vi "2D&3D Trajectory.vi"() -> ()   [LabVIEW 2014]
uses:
  <vilib>/LVH/AR Drone Toolkit/Decode NavData/Typedefs/NavData Demo.ctl
  <vilib>/Native 3D Graph/xcontrol/3DPC_SurfacePlot.xctl
  <vilib>/LVH/AR Drone Toolkit/AR Drone.lvlib
panel:
  out "3D Graph":refnum<class "Base Datatype.lvclass">[](xcontrol)
  in  "Setup Parameters":T1={"Drone IP address"="192.168.1.1", "Home IP address"="192.168.1.2", "Flight Mode"=enum."INDOOR MODE", "Mounted Hull"=enum."INDOOR HULL", "Video Camera"=1, "Max Altitude (m)"=3.0, "Max Pitch and Roll Angle (deg)"=10.0, "Max Vertical Speed (m/s)"=0.7, "Max Yaw Speed (deg/s)"=100.0} {"Video Camera" items=["Bottom Camera"=1, "Front Camera"=0, "Front in Bottom"=3, "Bottom in Front"=2]}
  out "NavData Out":T2={"control state"=enum."TRANS_LANDING", "battery percentage"=56, "pitch (deg)"=-0.108, "roll (deg)"=1.397, "yaw (deg)"=137.205, "altitude (cm)"=0, "vx (cm/s)?"=0.0, "vy (cm/s)?"=0.0, "vz (cm/s)?"=0.0, "detection cam type"=3}
  out "nav":errorcluster
  out "ctr":errorcluster
  out "XY Graph":cluster{"Y":dbl[], "Y":dbl[]}[](graph)
  in  "device ID":i32=3
  in  "Hover":bool
  in  "Take Off/Land":bool
  in  "Emergency Landing":bool
  in  "stop":bool=TRUE
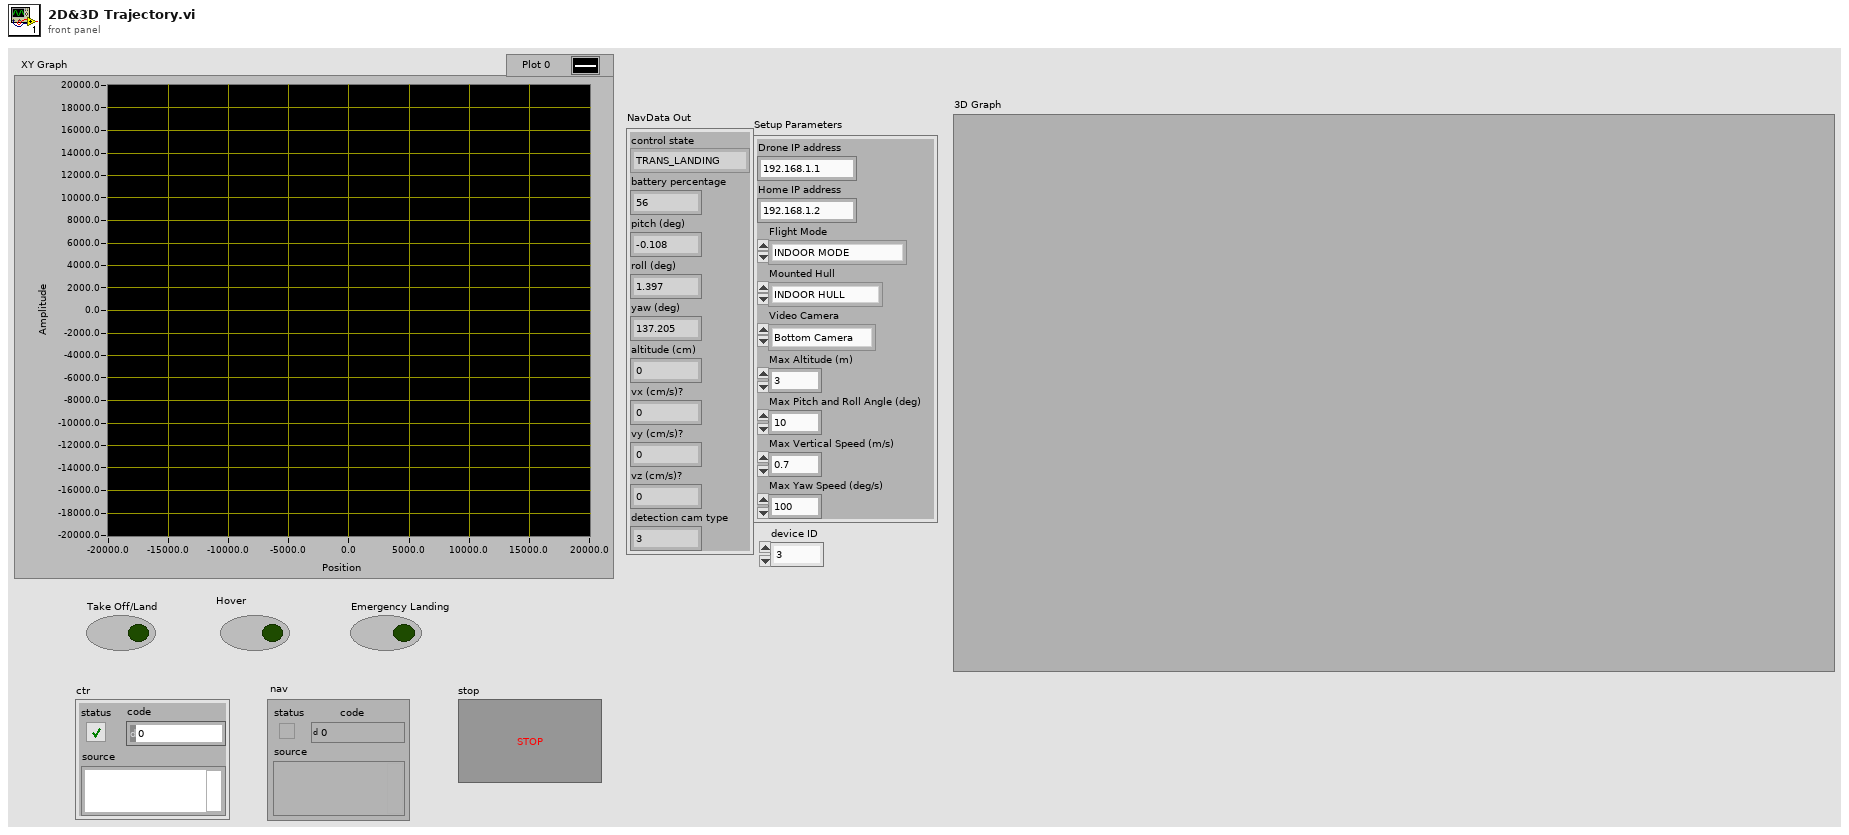
[diagram p1: front panel]
types:
  T1 = cluster{"Drone IP address":string, "Home IP address":string, "Flight Mode":enum8{"OUTDOOR MODE", "INDOOR MODE"}, "Mounted Hull":enum8{"OUTDOOR HULL", "INDOOR HULL"}, "Video Camera":u8, "Max Altitude (m)":sgl, "Max Pitch and Roll Angle (deg)":sgl, "Max Vertical Speed (m/s)":sgl, "Max Yaw Speed (deg/s)":sgl}
  T2 = typedef "AR Drone.lvlib/NavData Demo.ctl" = cluster{"control state":enum32{"DEFAULT", "INIT", "LANDING", "FLYING", "HOVERING", "TEST", "TRANS_TAKEOFF", "TRANS_GOTOFIX", "TRANS_LANDING"}, "battery percentage":u32, "pitch (deg)":sgl, "roll (deg)":sgl, "yaw (deg)":sgl, "altitude (cm)":u32, "vx (cm/s)?":sgl, "vy (cm/s)?":sgl, "vz (cm/s)?":sgl, "detection cam type":u32}
  T3 = typedef "AR Drone.lvlib/AR Drone Resource.ctl" = cluster{"UDP Control Connection":refnum<k16>, "UDP NavData Connection":refnum<k16>, "UDP Video Connection (Drone 1.0)":refnum<k16>, "TCP Video Connection (Drone 2.0)":refnum<k5>, "TCP Control Port Connection":refnum<k5>, "Drone IP address":string, "Drone Command Port":u16, "Drone NavData Port":u16, "Drone Vid Stream Port":u16, "Drone TCP Control Port":u16, "Home IP address":string, "Home Command Port":u16, "Home NavData Port":u16, "Home Vid Stream Port":u16, "Drone Version":i32, "Drone Index":i32, "Command Sequence":i32}
  T4 = cluster{"Roll":dbl, "Pitch":dbl, "Vertical Speed":dbl, "Yaw Speed":dbl}
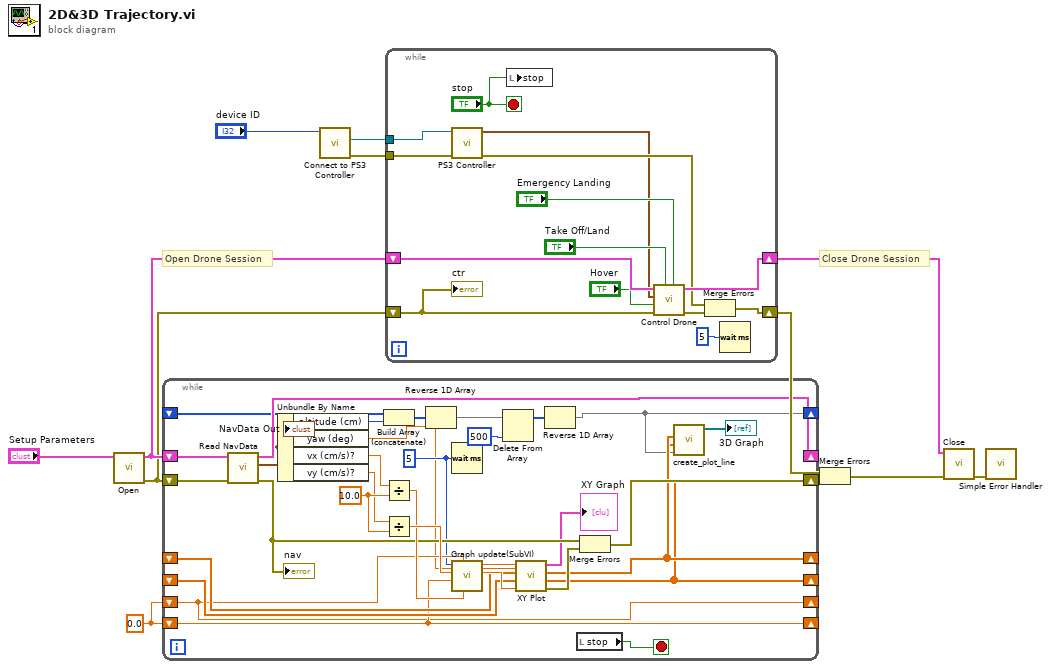
[diagram p0: block diagram]
diagram:
  w2 = 0.0
  # "Close Drone Session"
  # "Open Drone Session"
  n1 = call <vilib>:"Open.vi"("Setup Parameters"="Setup Parameters") -> ("error out"=w7:errorcluster, "AR Drone Resource"=w8:T3)  [unwired: 9 in]
  n2 = while {
    shift-right: [w41] -> _
    shift-left: w8 -> [w43]
    shift-right: [w28] -> w6
    shift-left: w7 -> [w42]
    shift-right: [w22] -> _
    shift-left: _ -> [w37]
    shift-right: [w21] -> _
    shift-left: _ -> [w38]
    shift-right: [w31] -> _
    shift-left: w2 -> [w31]
    shift-right: [w32] -> _
    shift-left: w2 -> [w32]
    shift-right: [w14] -> _
    shift-left: _ -> [w16]
    stop <- w44 stop-if-true
    w27 = u32 5 ("milliseconds to wait")
    w35 = sgl 10.0 ("y")
    n3 = call <vilib>:"Read NavData.vi"("error in (no error)"=w42, "AR Drone Resource"=w43) -> ("error out"=w29:errorcluster, "NavData Out"=w36:T2, "AR Drone Resource Out"=w41:T3)  [unwired: 7 in]
    "nav" <- w29
    "NavData Out" <- w36
    n4 = Unbundle By Name(w36) -> ("altitude (cm)"=w13:u32, "yaw (deg)"=w15:sgl, "vx (cm/s)?"=w26:sgl, "vy (cm/s)?"=w25:sgl)
    n5 = Build Array (concatenate)(w16, w13) -> (w19:u32[])
    n6 = Divide(x=w26, y=w35) -> (x/y=w33:sgl)
    n7 = Divide(x=w25, y=w35) -> (x/y=w34:sgl)
    n8 = Reverse 1D Array(array=w19) -> (reversed array=w18:u32[])
    n9 = Wait (ms)(milliseconds to wait=w27) -> ()  [unwired: 1 out]
    n10 = call "Graph update(SubVI).vi"("vy (cm/s)?"=w33, "Numeric 4"=w31, "Numeric in"=w32, "vx (cm/s)?"=w34, "milliseconds to wait"=w27) -> ("Numeric out"=w39:dbl, "Numeric 3"=w40:dbl)  [unwired: 5 in]
    n11 = Delete From Array(array=w18, index=500) -> (array with subset deleted=w17:u32[])  [unwired: 1 in, 1 out]
    n12 = call "XY Plot.vi"("X"=w40, "X array"=w37, "Y array"=w38, "Y"=w39, "Angle"=w15) -> ("XY Graph"=→"XY Graph":cluster{"Y":dbl[], "Y":dbl[]}[], "X array"=w22:dbl[], "Y array"=w21:dbl[], "error out"=w30:errorcluster)  [unwired: 1 out]
    n13 = Reverse 1D Array(array=w17) -> (reversed array=w14:u32[])
    n14 = local read "stop"() -> (w44:bool)
    n15 = Merge Errors(w29, w30) -> (w28:errorcluster)
    n16 = call <vilib>:"create_plot_line.vi"("z vector"=w14, "y vector"=w21, "x vector"=w22) -> ("plots out"=→"3D Graph":refnum<class "Base Datatype.lvclass">[])  [unwired: 2 in, 6 out]
  }
  n17 = call "Connect to PS3 Controller.vi"("device ID"="device ID") -> ("error out"=w5:errorcluster, "device ID 2"=w4:refnum<k1>)  [unwired: 7 in, 1 out]
  n18 = while {
    shift-right: [w54] -> w12
    shift-left: w8 -> [w58]
    shift-right: [w47] -> w9
    shift-left: w7 -> [w46]
    tunnel: w5 -> [w52]
    tunnel: w4 -> [w51]
    stop <- "stop" stop-if-true
    n19 = call "PS3 Controller.vi"("error in (no error)"=w52, "device ID"=w51) -> ("error out"=w48:errorcluster, "Control cluster"=w45:T4)  [unwired: 6 in, 2 out]
    n20 = local write "stop"("stop") -> ()
    n21 = call <vilib>:"Control Drone.vi"("Emergency Landing"="Emergency Landing", "Takeoff/Land"="Take Off/Land", "error in (no error)"=w46, "Hover"="Hover", "Control Cluster"=w45, "AR Drone Resource"=w58) -> ("error out"=w49:errorcluster, "AR Drone Resource Out"=w54:T3)  [unwired: 4 in]
    n22 = Merge Errors(w48, w49) -> (w47:errorcluster)
    n23 = Wait (ms)(milliseconds to wait=u32 5) -> ()  [unwired: 1 out]
    "ctr" <- w46
  }
  n24 = Merge Errors(w9, w6) -> (w10:errorcluster)
  n25 = call <vilib>:"Close.vi"("error in (no error)"=w10, "AR Drone Resource"=w12) -> ("error out"=w11:errorcluster)  [unwired: 9 in]
  n26 = call <vilib>:"Simple Error Handler.vi"("error in (no error)"=w11) -> ()  [unwired: 4 in, 5 out]
